vi "Get All PDP Data.vi"(0 "Power Distribution Panel (0)":u8, 11 "error in":errorcluster) -> (6 "PDP Data":T1, 15 "error out":errorcluster)   [LabVIEW 2014]
doc: "Returns the currents of the Power Distribution Panel (PDP) channels."
uses:
  PDP Data.ctl
  <vilib>/Rock Robotics/WPI/CAN/PDP/WPI_CAN_PDPGlobalOps.ctl
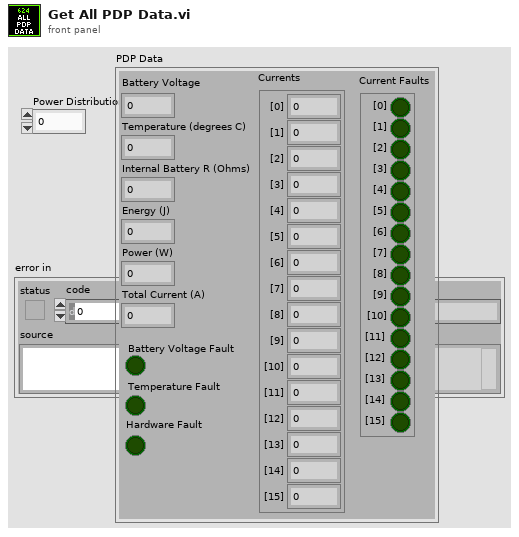
[diagram p1: front panel]
types:
  T1 = typedef "PDP Data.ctl" = cluster{"Battery Voltage":dbl, "Temperature (degrees C)":dbl, "Internal Battery R (Ohms)":dbl, "Energy (J)":dbl, "Power (W)":dbl, "Total Current (A)":dbl, "Battery Voltage Fault":bool, "Temperature Fault":bool, "Hardware Fault":bool, "Currents":cluster{"[0]":dbl, "[1]":dbl, "[2]":dbl, "[3]":dbl, "[4]":dbl, "[5]":dbl, "[6]":dbl, "[7]":dbl, "[8]":dbl, "[9]":dbl, "[10]":dbl, "[11]":dbl, "[12]":dbl, "[13]":dbl, "[14]":dbl, "[15]":dbl}, "Current Faults":cluster{"[0]":bool, "[1]":bool, "[2]":bool, "[3]":bool, "[4]":bool, "[5]":bool, "[6]":bool, "[7]":bool, "[8]":bool, "[9]":bool, "[10]":bool, "[11]":bool, "[12]":bool, "[13]":bool, "[14]":bool, "[15]":bool}}
  T2 = typedef "WPI_CAN_PDPGlobalOps.ctl" = enum16{"Write After Receive 0-5", "Write After Receive 6-11", "Write After Receive 12-15", "Write After Receive Energy", "Get All", "Get Commands", "Write Clear Sticky Faults Command", "Write Reset Energy Command", "Write Tare Currents Command", "Write Error", "Write After Receive Faults"}
  T3 = typedef "WPI_CAN_PDPGetAll.ctl" = cluster{"Channel Currents":dbl[], "Battery Voltage":dbl, "Temperature (degrees C)":dbl, "Internal Battery R (Ohms)":dbl, "Energy (J)":dbl, "Power (W)":dbl, "Total Current (A)":dbl, "CAN Error":errorcluster, "Current Faults":bool[], "Battery Voltage Fault":bool, "Temperature Fault":bool, "Hardware Fault":bool}
  T4 = cluster{"Channel Currents[0]":dbl, "Channel Currents[1]":dbl, "Channel Currents[2]":dbl, "Channel Currents[3]":dbl, "Channel Currents[4]":dbl, "Channel Currents[5]":dbl, "Channel Currents[6]":dbl, "Channel Currents[7]":dbl, "Channel Currents[8]":dbl, "Channel Currents[9]":dbl, "Channel Currents[10]":dbl, "Channel Currents[11]":dbl, "Channel Currents[12]":dbl, "Channel Currents[13]":dbl, "Channel Currents[14]":dbl, "Channel Currents[15]":dbl}
  T5 = cluster{"Current Faults[0]":bool, "Current Faults[1]":bool, "Current Faults[2]":bool, "Current Faults[3]":bool, "Current Faults[4]":bool, "Current Faults[5]":bool, "Current Faults[6]":bool, "Current Faults[7]":bool, "Current Faults[8]":bool, "Current Faults[9]":bool, "Current Faults[10]":bool, "Current Faults[11]":bool, "Current Faults[12]":bool, "Current Faults[13]":bool, "Current Faults[14]":bool, "Current Faults[15]":bool}
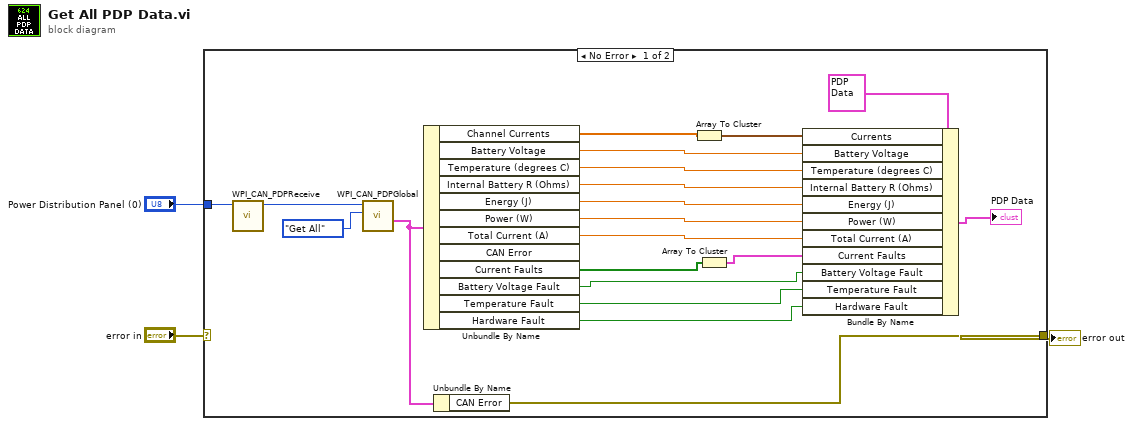
[diagram p0: block diagram]
diagram:
  n1 = case shown="No Error" "error in" {
    selector: "error in" -> [_ w24]
    tunnel: [w20 w24] -> w2
    tunnel: "Power Distribution Panel (0)" -> [w22 _]
    frame No Error {
      n2 = call <vilib>:"WPI_CAN_PDPReceive.vi"("Power Distribution Panel (0)"=w22) -> ("Power Distribution Panel Out"=w23:u8)  [unwired: 10 in]
      n3 = call <vilib>:"WPI_CAN_PDPGlobal.vi"("Operation"=WPI_CAN_PDPGlobalOps."Get All", "Power Distribution Panel (0)"=w23) -> ("Get All"=w19:T3)  [unwired: 7 in, 2 out]
      n4 = Unbundle By Name(w19) -> ("Channel Currents"=w7:dbl[], "Battery Voltage"=w16:dbl, "Temperature (degrees C)"=w15:dbl, "Internal Battery R (Ohms)"=w14:dbl, "Energy (J)"=w13:dbl, "Power (W)"=w12:dbl, "Total Current (A)"=w11:dbl, "Current Faults"=w6:bool[], "Battery Voltage Fault"=w10:bool, "Temperature Fault"=w9:bool, "Hardware Fault"=w8:bool)  [unwired: 1 out]
      n5 = Unbundle By Name(w19) -> ("CAN Error"=w20:errorcluster)
      n6 = Array To Cluster(array=w7) -> (cluster=w4:T4)
      n7 = Array To Cluster(array=w6) -> (cluster=w5:T5)
      n8 = Bundle By Name(cluster=T1 {"Battery Voltage"=0.0, "Temperature (degrees C)"=0.0, "Internal Battery R (Ohms)"=0.0, "Energy (J)"=0.0, "Power (W)"=0.0, "Total Current (A)"=0.0, "Battery Voltage Fault"=FALSE, "Temperature Fault"=FALSE, "Hardware Fault"=FALSE, "Currents"={"[0]"=0.0, "[1]"=0.0, "[2]"=0.0, "[3]"=0.0, "[4]"=0.0, "[5]"=0.0, "[6]"=0.0, "[7]"=0.0, "[8]"=0.0, "[9]"=0.0, "[10]"=0.0, "[11]"=0.0, "[12]"=0.0, "[13]"=0.0, "[14]"=0.0, "[15]"=0.0}, "Current Faults"={"[0]"=FALSE, "[1]"=FALSE, "[2]"=FALSE, "[3]"=FALSE, "[4]"=FALSE, "[5]"=FALSE, "[6]"=FALSE, "[7]"=FALSE, "[8]"=FALSE, "[9]"=FALSE, "[10]"=FALSE, "[11]"=FALSE, "[12]"=FALSE, "[13]"=FALSE, "[14]"=FALSE, "[15]"=FALSE}} ("PDP Data"), "Currents"=w4, "Battery Voltage"=w16, "Temperature (degrees C)"=w15, "Internal Battery R (Ohms)"=w14, "Energy (J)"=w13, "Power (W)"=w12, "Total Current (A)"=w11, "Current Faults"=w5, "Battery Voltage Fault"=w10, "Temperature Fault"=w9, "Hardware Fault"=w8) -> (→"PDP Data":T1)
    }
    frame Error {
    }
  }
  "error out" <- w2
